vi "Calculate time.vi"(8 "error in (no error)":errorcluster, 10 "Average time":dbl, 11 "Schedule in":refnum<class "Schedule.lvclass">) -> (0 "error out":errorcluster, 1 "Time":dbl, 2 "Number of scripts":u32, 3 "Schedule out":refnum<class "Schedule.lvclass">)   [LabVIEW 2020, in "CIRCUS_uServices.lvlib" / "Run Utilities.lvlib" / "Schedule.lvclass"]
doc: "Calculate number of scripts left in the shcedule and estimate time of the execution (in seconds) based on the average time"
uses:
  Schedule.lvclass
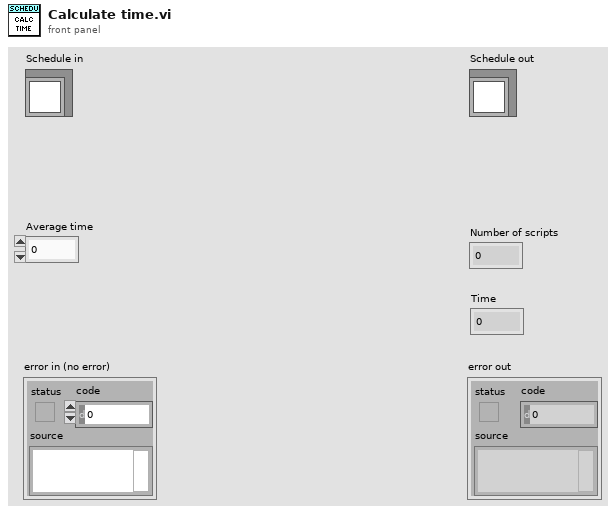
[diagram p1: front panel]
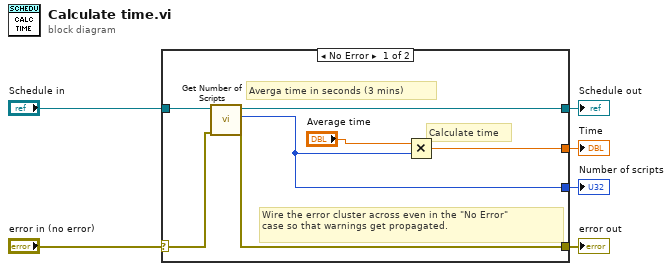
[diagram p0: block diagram]
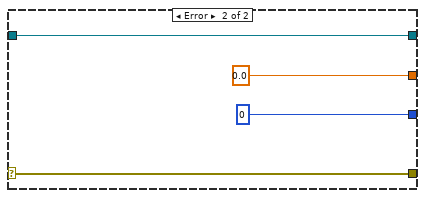
[diagram p2: hidden frame]
diagram:
  n1 = case shown="No Error" "error in (no error)" {
    selector: "error in (no error)" -> [w10 w17]
    tunnel: [w9 w17] -> w5
    tunnel: [w7 w16] -> w3
    tunnel: "Schedule in" -> [w11 w16]
    tunnel: [w13 0.0] -> w2
    tunnel: [w8 u32 0 ("y")] -> w1
    frame No Error {
      # "Wire the error cluster across even in the \"No Error\"\ncase so that warnings get propagated."
      # "Averga time in seconds (3 mins)"
      # "Calculate time"
      n2 = call-dynamic "Get Number of Scripts.vi"("error in (no error)"=w10, "Schedule in"=w11) -> ("error out"=w9:errorcluster, "No. of Scripts"=w8:u32, "Schedule out"=w7:refnum<class "Schedule.lvclass">)  [unwired: 7 in]
      n3 = Multiply(x="Average time", y=w8) -> (x*y=w13:dbl)
    }
    frame Error {
    }
  }
  "error out" <- w5
  "Schedule out" <- w3
  "Time" <- w2
  "Number of scripts" <- w1
